vi "Hallway to Room.vi"(11 "State in":cluster{"Hallway":string[], "Rooms":string[][]}) -> (1 "Moved?":bool, 2 "Best Cost":u64, 3 "State out":cluster{"Hallway":string[], "Rooms":string[][]})   [LabVIEW 2019, in "23.lvlib"]
uses:
  23.lvlib
  Between.vi
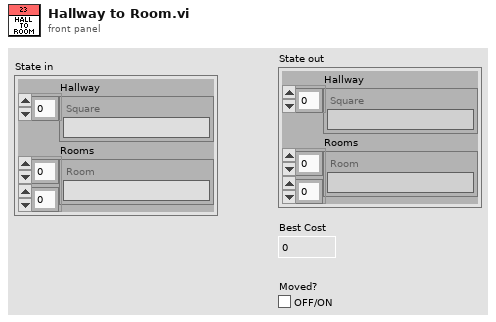
[diagram p1: front panel]
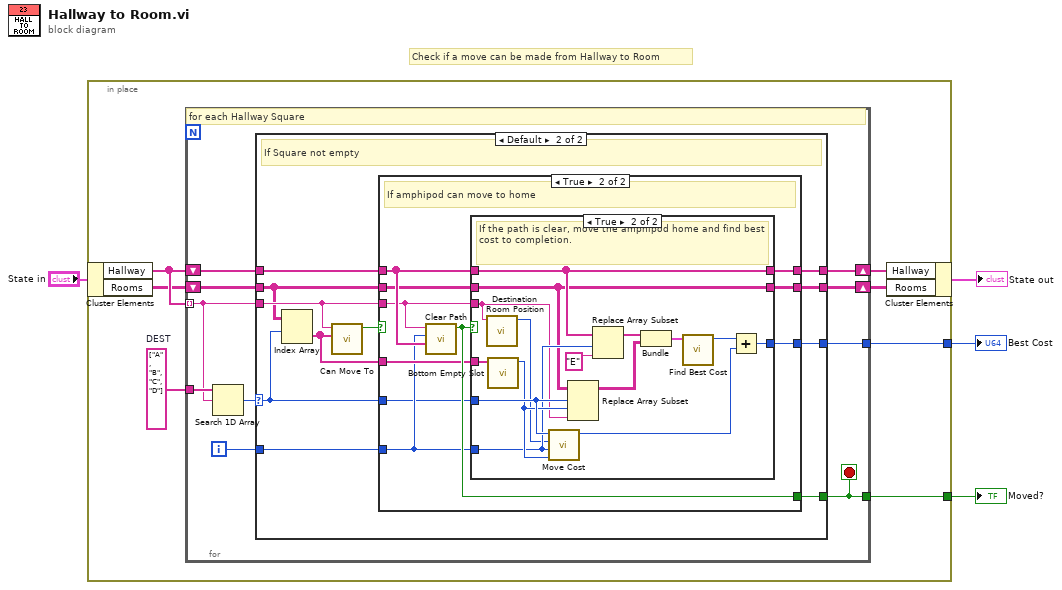
[diagram p0: block diagram]
diagram:
  # "Check if a move can be made from Hallway to Room"
  n1 = in-place {
    in-place-border: [w11] -> w4
    in-place-border: [w10] -> w3
    w9 = string[] ["A", "B", "C", "D"]  # DEST
    n2 = in-place-cluster #1("State in") -> ("Hallway"=w8:string[], "Rooms"=w7:string[][])
    n3 = for {
      tunnel: w8 -> [w12] mode=indexing
      tunnel: w9 -> [w21]
      tunnel: [w17] -> w10
      tunnel: [w16] -> w11
      shift-right: [w15] -> w6
      shift-left: w8 -> [w18]
      shift-right: [w14] -> w5
      shift-left: w7 -> [w20]
      i -> [w19]
      stop <- w16 stop-if-true
      # "for each Hallway Square"
      n4 = Search 1D Array(1D array=w21, element=w12) -> (index of element=w13:i32)  [unwired: 1 in]
      n5 = case shown="Default" w13 {
        selector: w13 -> [_ w26]
        tunnel: w19 -> [_ w34]
        tunnel: w18 -> [w23 w33]
        tunnel: w12 -> [_ w32]
        tunnel: w20 -> [w22 w30]
        tunnel: [_ w29] -> w16
        tunnel: [_ w27] -> w17
        tunnel: [w23 w25] -> w15
        tunnel: [w22 w24] -> w14
        frame -1 {
          # "if position empty try next position"
        }
        frame Default {
          # "If Square not empty"
          n6 = Index Array(array=w30, index (row)=w26) -> (element=w28:string[])  [unwired: 1 in]
          n7 = call "Can Move To.vi"("Room"=w28, "Amphipod Type"=w32) -> ("Can Move To?"=w31:bool)  [unwired: 9 in]
          n8 = case shown="True" w31 {
            tunnel: w34 -> [_ w41]
            tunnel: w33 -> [w36 w46]
            tunnel: w32 -> [_ w44]
            tunnel: w30 -> [w35 w45]
            tunnel: [_ w43] -> w29
            tunnel: w28 -> [_ w42]
            tunnel: [_ w40] -> w27
            tunnel: w26 -> [_ w39]
            tunnel: [w36 w38] -> w25
            tunnel: [w35 w37] -> w24
            frame False {
              # "If amphipod in position can't move home, try next position"
            }
            frame True {
              # "If amphipod can move to home"
              n9 = call "Clear Path.vi"("Hallway"=w46, "Hallway Position"=w41, "Room"=w44) -> ("Clear Path?"=w43:bool)  [unwired: 8 in]
              n10 = case shown="True" w43 {
                tunnel: w46 -> [w48 w50]
                tunnel: w45 -> [w47 w49]
                tunnel: w44 -> [_ w51]
                tunnel: w42 -> [_ w63]
                tunnel: w41 -> [_ w53]
                tunnel: [_ w58] -> w40
                tunnel: w39 -> [_ w55]
                tunnel: [w48 w50] -> w38
                tunnel: [w47 w49] -> w37
                frame False {
                  # "if path is not clear, try next position"
                }
                frame True {
                  # "If the path is clear, move the amphipod home and find best cost to completion."
                  n11 = call "Destination Room Position.vi"("Amphipod Type"=w51) -> ("Destination Room Position"=w52:i32)  [unwired: 10 in]
                  n12 = call "Bottom Empty Slot.vi"("Room"=w63) -> ("Slot"=w54:i32)  [unwired: 10 in]
                  n13 = call "Move Cost.vi"("Room Slot"=w54, "Destination Position"=w53, "Source Position"=w52, "Amphipod Type Index"=w55) -> ("Move Cost"=w57:u64)  [unwired: 7 in]
                  n14 = Replace Array Subset(array=w49, new element=w51, index (row)=w55, index (col)=w54) -> (w60:string[][])
                  n15 = Replace Array Subset(array=w50, new element="E" ("y"), index=w53) -> (w61:string[])
                  n16 = Bundle("Hallway"=w61, "Rooms"=w60) -> (w62:cluster{"Hallway":string[], "Rooms":string[][]})  [unwired: 1 in]
                  n17 = call "Find Best Cost.vi"("State"=w62) -> ("Best Cost"=w59:u64)  [unwired: 10 in]
                  n18 = Add(x=w59, y=w57) -> (x+y=w58:u64)
                }
              }
            }
          }
        }
      }
    }
    n19 = in-place-cluster #1("Hallway"=w6, "Rooms"=w5) -> (→"State out":cluster{"Hallway":string[], "Rooms":string[][]})
  }
  "Moved?" <- w4
  "Best Cost" <- w3
